vi "BITMOD.vi"(1 "Data":u8 format="%x", 2 "Mask":u8 format="%x", 3 "Address":u8 format="%x", 4 "SPI Config In":T1) -> (0 "SPI Config Out":T1)   [LabVIEW 2019]
uses:
  SPI/SPI Config.ctl
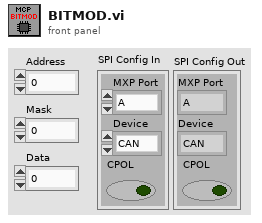
[diagram p1: front panel]
types:
  T1 = typedef "SPI Config.ctl" = cluster{"MXP Port":enum16{"A", "B"}, "Device":enum16{"CAN", "ENC", "IMU1", "IMU2"}, "CPOL":bool}
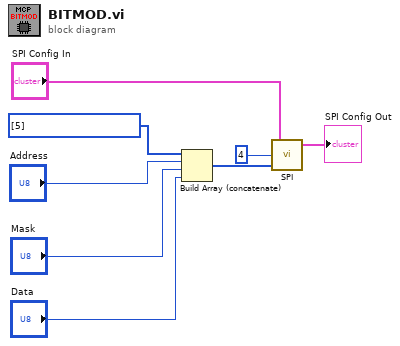
[diagram p0: block diagram]
diagram:
  n1 = Build Array (concatenate)(u8[] [5] ("Frames to Write"), "Address", "Mask", "Data") -> (w4:u8[])
  n2 = call "SPI.vi"("Data to Write"=w4, "Frames to Write"=u8 4, "SPI Config In"="SPI Config In") -> ("SPI Config Out"=→"SPI Config Out":T1)  [unwired: 2 out]
